vi "Open Recording File.vi"(8 "error in (no error)":errorcluster, 11 "AcquireTraces In":refnum<class "AcquireTraces.lvclass">) -> (0 "error out":errorcluster, 3 "AcquireTraces Out":refnum<class "AcquireTraces.lvclass">)   [LabVIEW 2010, in "AcquireTraces.lvclass"]
uses:
  AcquireTraces/AcquireTraces.lvclass
  AcquireTraces/AcquireTraces.lvclass/AcquireTraces.ctl
  HDF5Tools/LabView/Create Dataset 2D Integer.vi
  HDF5Tools/LabView/HDF5Tools.lvlib
  Program Files/National Instruments/LabVIEW 2010/resource/objmgr/daqmx.rc
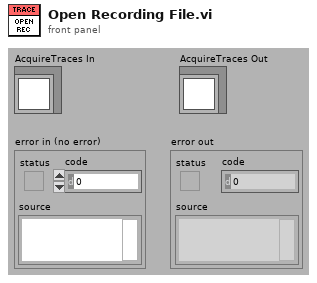
[diagram p1: front panel]
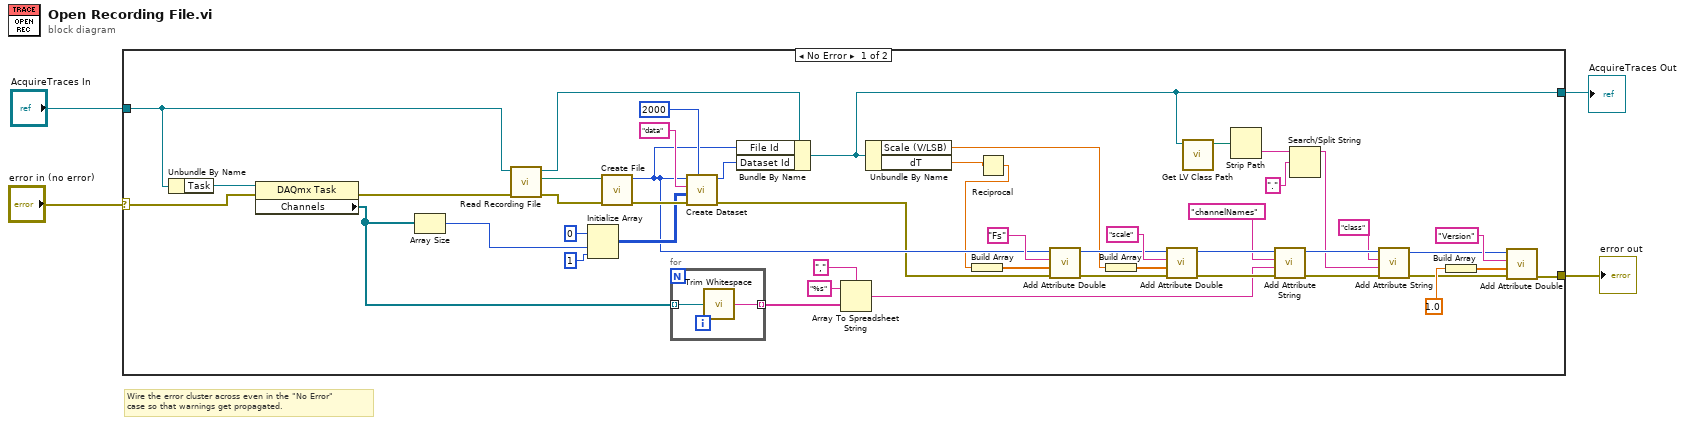
[diagram p0: block diagram]
diagram:
  # "Wire the error cluster across even in the \"No Error\"\ncase so that warnings get propagated."
  n1 = case shown="No Error" "error in (no error)" {
    selector: "error in (no error)" -> [w27 w56]
    tunnel: [w5 w56] -> w3
    tunnel: [w16 w55] -> w2
    tunnel: "AcquireTraces In" -> [w42 w55]
    frame No Error {
      n2 = Unbundle By Name(w42) -> ("Task"=w28:refnum<k21>)
      n3 = property class="DAQmx Task"(reference=w28, error in=w27) -> (error out=w25:errorcluster, "Channels"=w21:refnum<k21>[])  [unwired: 1 out]
      n4 = Array Size(array=w21) -> (size(s)=w26:i32)
      n5 = call-dynamic "Read Recording File.vi"("error in (no error)"=w25, "AcquistionObject in"=w42) -> ("error out"=w44:errorcluster, "Recording File"=w45:path, "AcquistionObject out"=w43:refnum<class "AcquireTraces.lvclass">)  [unwired: 7 in]
      n6 = Initialize Array(0, w26, 1 ("dimension size")) -> (w47:i32[][])
      n7 = call "Create File.vi"("Error in"=w44, "File Name"=w45) -> ("Error out"=w52:errorcluster, "file_id"=w24:i32)  [unwired: 6 in]
      n8 = for {
        tunnel: w21 -> [w53] mode=indexing
        tunnel: [w54] -> w34 mode=indexing
        n9 = call <vilib>:"Trim Whitespace.vi"("string"=w53) -> ("trimmed string"=w54:string)  [unwired: 1 in]
      }
      n10 = call-poly "Create Dataset.vi"("Chunk size"=2000, "error in (no error)"=w52, "Datatype"=w47, "Dataset name"="data", "Location id in"=w24) -> ("error out"=w22:errorcluster, "Dataset id"=w46:i32)  [unwired: 5 in]
      n11 = Bundle By Name(cluster=w43, "File Id"=w24, "Dataset Id"=w46) -> (w16:refnum<class "AcquireTraces.lvclass">)
      n12 = Array To Spreadsheet String(delimiter (Tab)=",", array=w34, 3:"%s" ("format string")) -> (spreadsheet string=w29:string)
      n13 = Unbundle By Name(w16) -> ("Scale (V/LSB)"=w23:dbl, "dT"=w7:dbl)
      n14 = Reciprocal(x=w7) -> (1/x=w6:dbl)
      n15 = Build Array(w6) -> (w40:dbl[])
      n16 = call "Add Attribute Double.vi"("error in (no error)"=w22, "data"=w40, "Attribute name"="Fs", "loc_id"=w24) -> ("error out"=w39:errorcluster, "loc_id_out"=w31:i32)  [unwired: 6 in]
      n17 = Build Array(w23) -> (w37:dbl[])
      n18 = call "Add Attribute Double.vi"("error in (no error)"=w39, "data"=w37, "Attribute name"="scale", "loc_id"=w31) -> ("error out"=w33:errorcluster, "loc_id_out"=w32:i32)  [unwired: 6 in]
      n19 = call <vilib>:"Get LV Class Path.vi"("object"=w16) -> ("class path"=w19:path)  [unwired: 9 in, 1 out]
      n20 = Strip Path(path=w19) -> (name=w18:string)  [unwired: 1 out]
      n21 = call "Add Attribute String.vi"("error in (no error)"=w33, "Attribute data"=w29, "Attribute name"="channelNames", "loc_id"=w32) -> ("error out"=w14:errorcluster, "loc_id_out"=w20:i32)  [unwired: 6 in]
      n22 = Search/Split String(string=w18, search string/char (-)=".") -> (substring before match=w13:string)  [unwired: 1 in, 2 out]
      n23 = call "Add Attribute String.vi"("error in (no error)"=w14, "Attribute data"=w13, "Attribute name"="class", "loc_id"=w20) -> ("error out"=w10:errorcluster, "loc_id_out"=w8:i32)  [unwired: 6 in]
      n24 = Build Array(1.0) -> (w9:dbl[])
      n25 = call "Add Attribute Double.vi"("error in (no error)"=w10, "data"=w9, "Attribute name"="Version", "loc_id"=w8) -> ("error out"=w5:errorcluster)  [unwired: 6 in, 1 out]
    }
    frame Error {
    }
  }
  "error out" <- w3
  "AcquireTraces Out" <- w2
